vi "System Status Display.vi"(0 "InterfaceData":T1 {"GenEast"."TotalFuel(L)" format="%.2f"; "GenEast"."FuelRate(L/H)" format="%.2f"; "GenEast"."ApparentPower(VA)" format="%.2f"; "GenEast"."BattVoltage(V)" format="%.2f"; "GenEast"."Freq(Hz)" format="%.2f"; "GenEast"."RunHours(hr)" format="%.2f"; "GenEast"."PowerFactor" format="%.2f"; "GenEast"."ReactivePower(VAR)" format="%.2f"; "GenEast"."ActivePower(W)" format="%.2f"; "GenWest"."TotalFuel(L)" format="%.2f"; "GenWest"."FuelRate(L/H)" format="%.2f"; "GenWest"."ApparentPower(VA)" format="%.2f"; "GenWest"."BattVoltage(V)" format="%.2f"; "GenWest"."Freq(Hz)" format="%.2f"; "GenWest"."RunHours(hr)" format="%.2f"; "GenWest"."PowerFactor" format="%.2f"; "GenWest"."ReactivePower(VAR)" format="%.2f"; "GenWest"."ActivePower(W)" format="%.2f"; "Converter Alarms 2" format="%016b"; "Converter Faults 2" format="%016b"; "Controller Faults" format="%016b"; "System Status" format="%016b"; "Converter Alarms 1" format="%016b"; "Converter Faults 1" format="%016b"; "Solar Faults" format="%016b"; "ES Rack 10 Alarms" format="%016b"; "ES Rack 9 Alarms" format="%016b"; "ES Rack 8 Alarms" format="%016b"; "ES Rack 7 Alarms" format="%016b"; "ES Rack 6 Alarms" format="%016b"; "ES Rack 5 Alarms" format="%016b"; "ES Rack 4 Alarms" format="%016b"; "ES Rack 3 Alarms" format="%016b"; "ES Rack 2 Alarms" format="%016b"; "ES Rack 1 Alarms" format="%016b"; "ES System Alarms" format="%016b"; "System Faults" format="%016b"; "ES Rack 10 Faults" format="%016b"; "ES Rack 9 Faults" format="%016b"; "ES Rack 8 Faults" format="%016b"; "ES Rack 7  Faults" format="%016b"; "ES Rack 6 Faults" format="%016b"; "ES Rack 5 Faults" format="%016b"; "ES Rack 4 Faults" format="%016b"; "ES Rack 3 Faults" format="%016b"; "ES Rack 2 Faults" format="%016b"; "ES Rack 1 Faults" format="%016b"; "ES System Faults" format="%016b"}, 5 "Connection Error":bool, 11 "Error In":errorcluster) -> (1 "FPGA Version":string, 2 "RT Version":string, 3 "Converter Version":string, 4 "System Status":string, 6 "System Status Data":bool[](array[boolean]), 8 "Gen Status Data":bool[](array[boolean]), 15 "Error Out":errorcluster)   [LabVIEW 2014]
uses:
  Controls/Interface Data.ctl
  Controls/Gen Data.ctl
panel:
  out "InterfaceData":T1 {"GenEast"."TotalFuel(L)" format="%.2f"; "GenEast"."FuelRate(L/H)" format="%.2f"; "GenEast"."ApparentPower(VA)" format="%.2f"; "GenEast"."BattVoltage(V)" format="%.2f"; "GenEast"."Freq(Hz)" format="%.2f"; "GenEast"."RunHours(hr)" format="%.2f"; "GenEast"."PowerFactor" format="%.2f"; "GenEast"."ReactivePower(VAR)" format="%.2f"; "GenEast"."ActivePower(W)" format="%.2f"; "GenWest"."TotalFuel(L)" format="%.2f"; "GenWest"."FuelRate(L/H)" format="%.2f"; "GenWest"."ApparentPower(VA)" format="%.2f"; "GenWest"."BattVoltage(V)" format="%.2f"; "GenWest"."Freq(Hz)" format="%.2f"; "GenWest"."RunHours(hr)" format="%.2f"; "GenWest"."PowerFactor" format="%.2f"; "GenWest"."ReactivePower(VAR)" format="%.2f"; "GenWest"."ActivePower(W)" format="%.2f"; "Converter Alarms 2" format="%016b"; "Converter Faults 2" format="%016b"; "Controller Faults" format="%016b"; "System Status" format="%016b"; "Converter Alarms 1" format="%016b"; "Converter Faults 1" format="%016b"; "Solar Faults" format="%016b"; "ES Rack 10 Alarms" format="%016b"; "ES Rack 9 Alarms" format="%016b"; "ES Rack 8 Alarms" format="%016b"; "ES Rack 7 Alarms" format="%016b"; "ES Rack 6 Alarms" format="%016b"; "ES Rack 5 Alarms" format="%016b"; "ES Rack 4 Alarms" format="%016b"; "ES Rack 3 Alarms" format="%016b"; "ES Rack 2 Alarms" format="%016b"; "ES Rack 1 Alarms" format="%016b"; "ES System Alarms" format="%016b"; "System Faults" format="%016b"; "ES Rack 10 Faults" format="%016b"; "ES Rack 9 Faults" format="%016b"; "ES Rack 8 Faults" format="%016b"; "ES Rack 7  Faults" format="%016b"; "ES Rack 6 Faults" format="%016b"; "ES Rack 5 Faults" format="%016b"; "ES Rack 4 Faults" format="%016b"; "ES Rack 3 Faults" format="%016b"; "ES Rack 2 Faults" format="%016b"; "ES Rack 1 Faults" format="%016b"; "ES System Faults" format="%016b"}
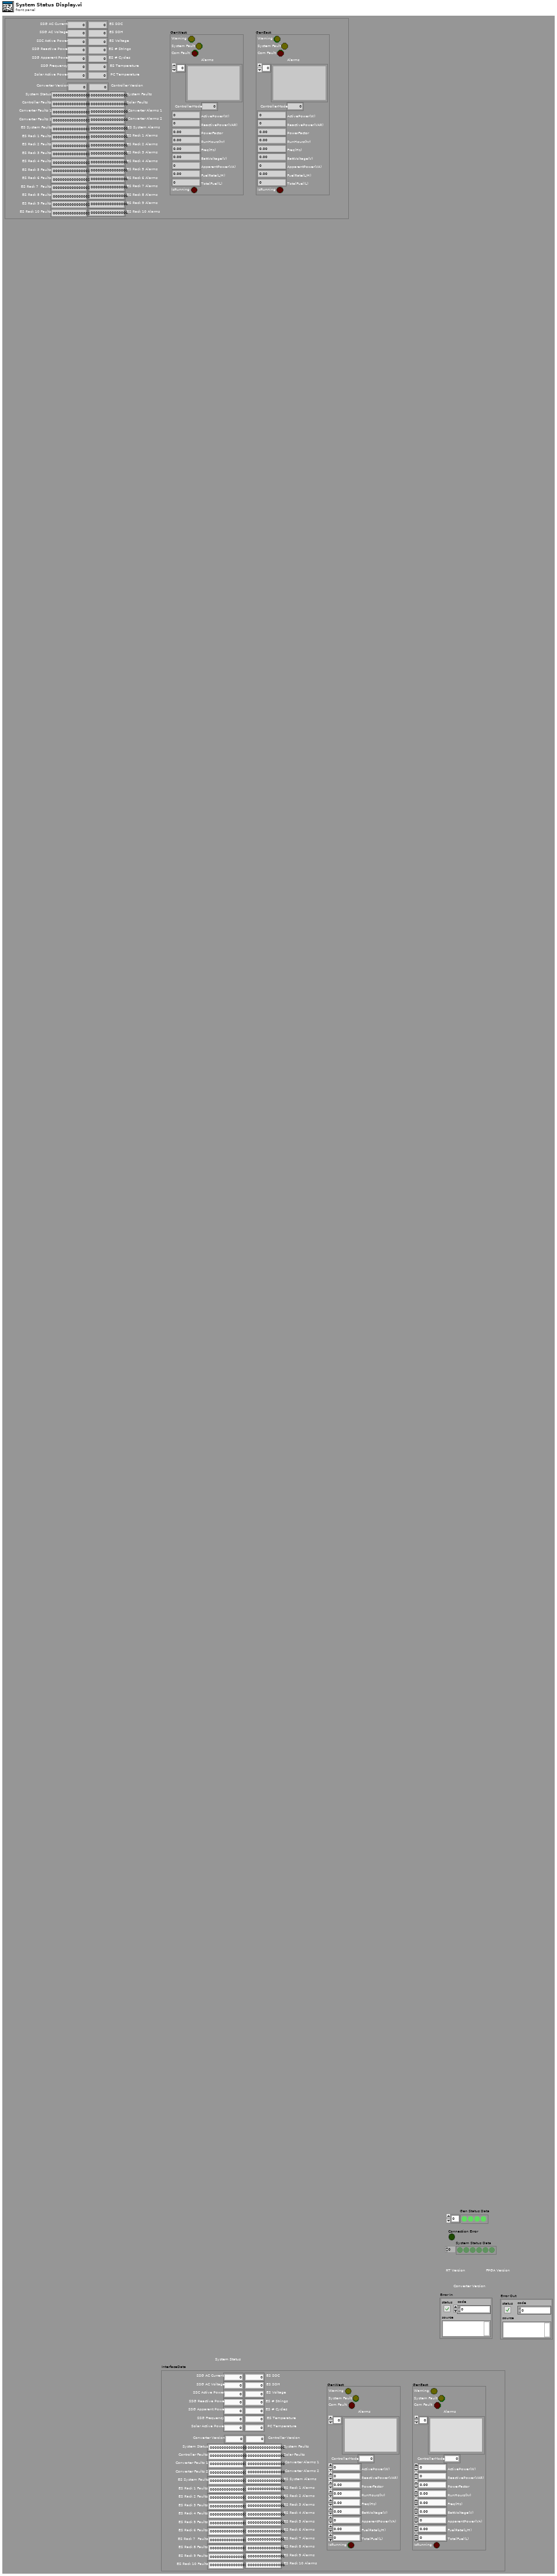
[diagram p1: front panel]
types:
  T1 = typedef "Interface Data.ctl" = cluster{"SSG AC Current":i16, "SSG AC Voltage":i16, "SSC Active Power":i16, "SSG Reactive Power":i16, "SSG Apparent Power":i16, "SSG Frequency":i16, "ES SOC":i16, "ES SOH":i16, "ES Voltage":i16, "ES # Strings":i16, "ES # Cycles":i16, "ES Temperature":i16, "PC Temperature":i16, "Solar Active Power":i16, "Converter Version":i16, "Controller Version":i16, "System Status":i16, "System Faults":i16, "Controller Faults":i16, "ES System Faults":i16, "ES System Alarms":i16, "Converter Faults 1":i16, "Converter Faults 2":i16, "Converter Alarms 1":i16, "Converter Alarms 2":i16, "Solar Faults":i16, "ES Rack 1 Faults":i16, "ES Rack 2 Faults":i16, "ES Rack 3 Faults":i16, "ES Rack 4 Faults":i16, "ES Rack 5 Faults":i16, "ES Rack 6 Faults":i16, "ES Rack 7  Faults":i16, "ES Rack 8 Faults":i16, "ES Rack 9 Faults":i16, "ES Rack 10 Faults":i16, "ES Rack 1 Alarms":i16, "ES Rack 2 Alarms":i16, "ES Rack 3 Alarms":i16, "ES Rack 4 Alarms":i16, "ES Rack 5 Alarms":i16, "ES Rack 6 Alarms":i16, "ES Rack 7 Alarms":i16, "ES Rack 8 Alarms":i16, "ES Rack 9 Alarms":i16, "ES Rack 10 Alarms":i16, "GenWest":T2, "GenEast":T2}
  T2 = typedef "Gen Data.ctl" = cluster{"Warning":bool, "System Fault":bool, "Com Fault":bool, "Alarms":string[], "ControllerMode":u16, "ActivePower(W)":i32, "ReactivePower(VAR)":i32, "PowerFactor":dbl, "RunHours(hr)":dbl, "Freq(Hz)":dbl, "BattVoltage(V)":dbl, "ApparentPower(VA)":i32, "FuelRate(L/H)":dbl, "TotalFuel(L)":u32, "IsRunning":bool}
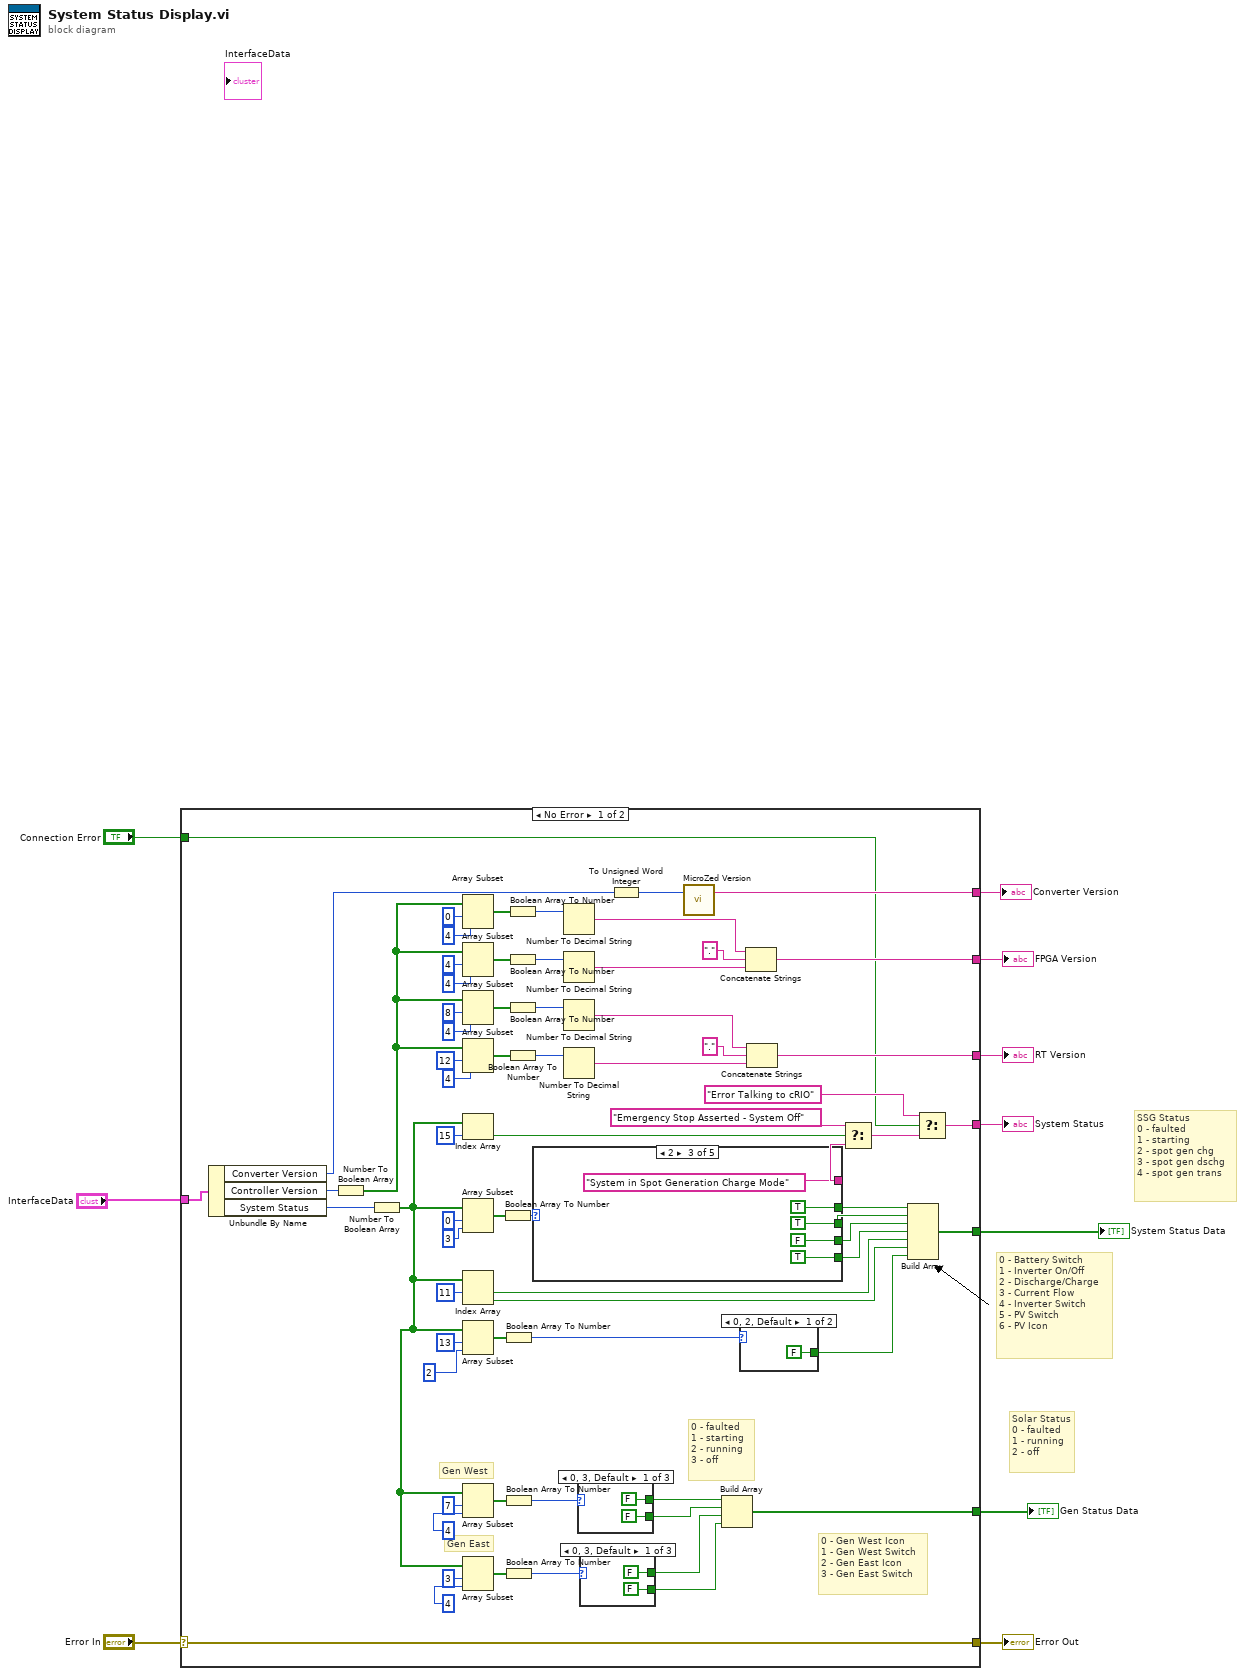
[diagram p0: block diagram]
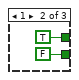
[diagram p2: hidden frame]
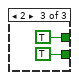
[diagram p3: hidden frame]
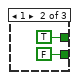
[diagram p4: hidden frame]
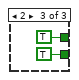
[diagram p5: hidden frame]
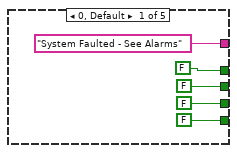
[diagram p6: hidden frame]
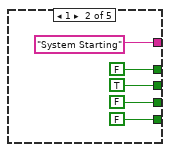
[diagram p7: hidden frame]
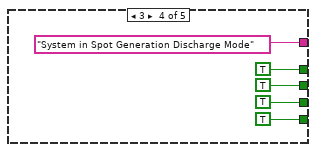
[diagram p8: hidden frame]
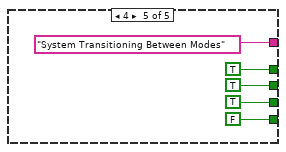
[diagram p9: hidden frame]
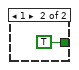
[diagram p10: hidden frame]
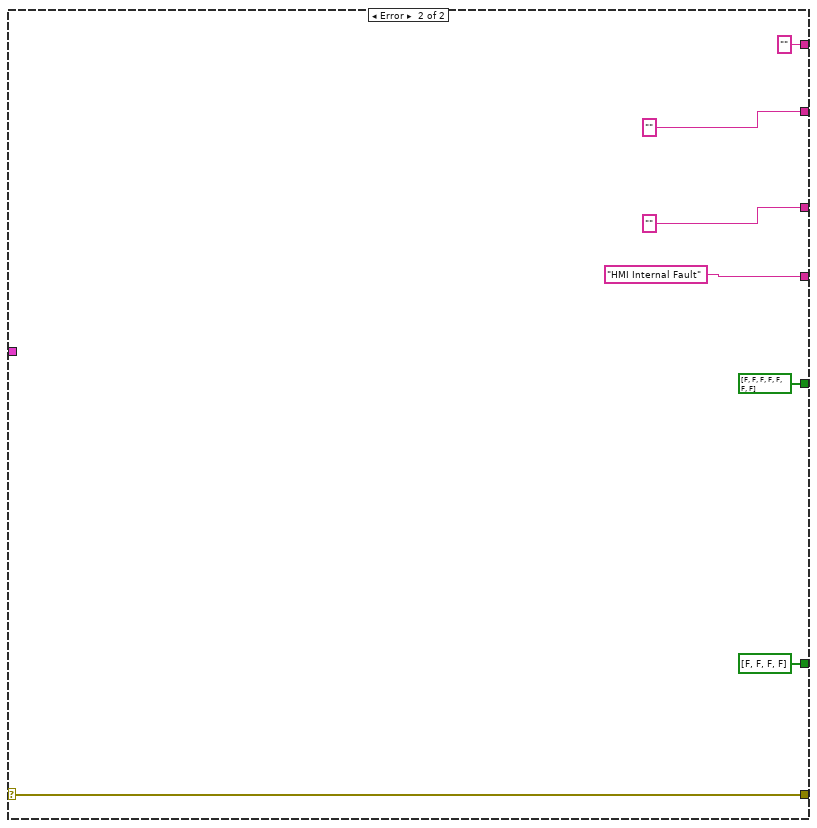
[diagram p11: hidden frame]
diagram:
  # "0 - Battery Switch\n1 - Inverter On/Off\n2 - Discharge/Charge\n3 - Current Flow\n4 - Inverter Switch\n5 - PV Switch\n6 - PV Icon"
  # "Solar Status\n0 - faulted\n1 - running\n2 - off"
  # "SSG Status\n0 - faulted\n1 - starting\n2 - spot gen chg\n3 - spot gen dschg\n4 - spot gen trans"
  n1 = case shown="No Error" "Error In" {
    selector: "Error In" -> [w47 w127]
    tunnel: [w47 w127] -> w9
    tunnel: "InterfaceData" -> [w81 _]
    tunnel: [w49 "HMI Internal Fault" ("System Status")] -> w8
    tunnel: [w51 ""] -> w7
    tunnel: [w50 ""] -> w6
    tunnel: "Connection Error" -> [w13 _]
    tunnel: [w29 bool[] [FALSE, FALSE, FALSE, FALSE]] -> w4
    tunnel: [w21 bool[] [FALSE, FALSE, FALSE, FALSE, FALSE, FALSE, FALSE]] -> w3
    tunnel: [w18 "" ("Version String")] -> w2
    frame No Error {
      # "Gen East"
      # "Gen West"
      # "0 - Gen West Icon\n1 - Gen West Switch\n2 - Gen East Icon\n3 - Gen East Switch"
      # "0 - faulted\n1 - starting\n2 - running \n3 - off"
      n2 = Unbundle By Name(w81) -> ("Converter Version"=w20:i16, "Controller Version"=w75:i16, "System Status"=w11:i16)
      n3 = Number To Boolean Array(number=w75) -> (Boolean array=w72:bool[])
      n4 = Number To Boolean Array(number=w11) -> (Boolean array=w30:bool[])
      n5 = Array Subset(array=w72, index=0, length=4) -> (w65:bool[])
      n6 = Array Subset(array=w72, index=4, length=4) -> (w62:bool[])
      n7 = Array Subset(array=w72, index=8, length=4) -> (w63:bool[])
      n8 = Array Subset(array=w72, index=12, length=4) -> (w64:bool[])
      n9 = Index Array(array=w30, index=15) -> (element=w14:bool)
      n10 = Array Subset(array=w30, index=0, length=3) -> (w17:bool[])
      n11 = Index Array(array=w30, index #1=11 ("index")) -> (element #1=w24:bool, element #2=w23:bool)  [unwired: 1 in]
      n12 = Array Subset(array=w30, index=13, length=2 ("index")) -> (w76:bool[])
      n13 = Array Subset(array=w30, index=7, length=4) -> (w36:bool[])
      n14 = Array Subset(array=w30, index=3, length=4) -> (w33:bool[])
      n15 = Boolean Array To Number(Boolean array=w17) -> (number=w16:u32)
      n16 = Boolean Array To Number(Boolean array=w76) -> (number=w15:u32)
      n17 = Boolean Array To Number(Boolean array=w36) -> (number=w32:u8)
      n18 = Boolean Array To Number(Boolean array=w33) -> (number=w31:u8)
      n19 = Boolean Array To Number(Boolean array=w65) -> (number=w61:u32)
      n20 = Boolean Array To Number(Boolean array=w62) -> (number=w60:u32)
      n21 = Boolean Array To Number(Boolean array=w63) -> (number=w59:u32)
      n22 = Boolean Array To Number(Boolean array=w64) -> (number=w58:u32)
      n23 = case shown="2" w16 {
        tunnel: [FALSE TRUE TRUE TRUE TRUE] -> w27
        tunnel: [FALSE FALSE FALSE TRUE TRUE] -> w26
        tunnel: [FALSE FALSE TRUE TRUE FALSE] -> w25
        tunnel: ["System Faulted - See Alarms" ("System Status") "System Starting" ("System Status") "System in Spot Generation Charge Mode" ("System Status") "System in Spot Generation Discharge Mode" ("System Status") "System Transitioning Between Modes" ("System Status")] -> w46
        tunnel: [FALSE FALSE TRUE TRUE TRUE] -> w28
        frame 0, Default {
        }
        frame 1 {
        }
        frame 2 {
        }
        frame 3 {
        }
        frame 4 {
        }
      }
      n24 = Number To Decimal String(number=w61) -> (decimal integer string=w52:string)  [unwired: 1 in]
      n25 = Number To Decimal String(number=w60) -> (decimal integer string=w54:string)  [unwired: 1 in]
      n26 = Number To Decimal String(number=w59) -> (decimal integer string=w55:string)  [unwired: 1 in]
      n27 = Number To Decimal String(number=w58) -> (decimal integer string=w57:string)  [unwired: 1 in]
      n28 = case shown="0, 3, Default" w32 {
        tunnel: [FALSE TRUE TRUE] -> w42
        tunnel: [FALSE FALSE TRUE] -> w41
        frame 0, 3, Default {
        }
        frame 1 {
        }
        frame 2 {
        }
      }
      n29 = case shown="0, 3, Default" w31 {
        tunnel: [FALSE TRUE TRUE] -> w40
        tunnel: [FALSE FALSE TRUE] -> w39
        frame 0, 3, Default {
        }
        frame 1 {
        }
        frame 2 {
        }
      }
      n30 = To Unsigned Word Integer(number=w20) -> (unsigned 16bit integer=w19:u16)
      n31 = call "MicroZed Version.vi"("Version Numeric"=w19) -> ("Version String"=w18:string)  [unwired: 2 in]
      n32 = Build Array(w42, w41, w40, w39) -> (w29:bool[])
      n33 = case shown="0, 2, Default" w15 {
        tunnel: [FALSE TRUE] -> w22
        frame 0, 2, Default {
        }
        frame 1 {
        }
      }
      n34 = Concatenate Strings(w52, "." ("string"), w54) -> (w51:string)
      n35 = Concatenate Strings(w55, "." ("string"), w57) -> (w50:string)
      n36 = Select(t="Emergency Stop Asserted - System Off", s=w14, f=w46) -> (s? t:f=w44:string)
      n37 = Build Array(w28, w27, w26, w25, w24, w23, w22) -> (w21:bool[])
      n38 = Select(t="Error Talking to cRIO" ("string"), s=w13, f=w44) -> (s? t:f=w49:string)
    }
    frame Error {
    }
  }
  "Error Out" <- w9
  "System Status" <- w8
  "System Status Data" <- w3
  "RT Version" <- w6
  "FPGA Version" <- w7
  "Gen Status Data" <- w4
  "Converter Version" <- w2
